vi "Window Graph.vi"(8 "error in (no error)":errorcluster, 9 "Window":dbl[unit]=10.0, 10 "Graph ref":refnum<vi>, 11 "Readable in":refnum<class "Readable.lvclass">) -> (0 "error out":errorcluster, 3 "Readable out":refnum<class "Readable.lvclass">)   [LabVIEW 2012, in "Readable.lvclass"]
uses:
  Readable.lvclass
  Readable.lvclass/Readable.ctl
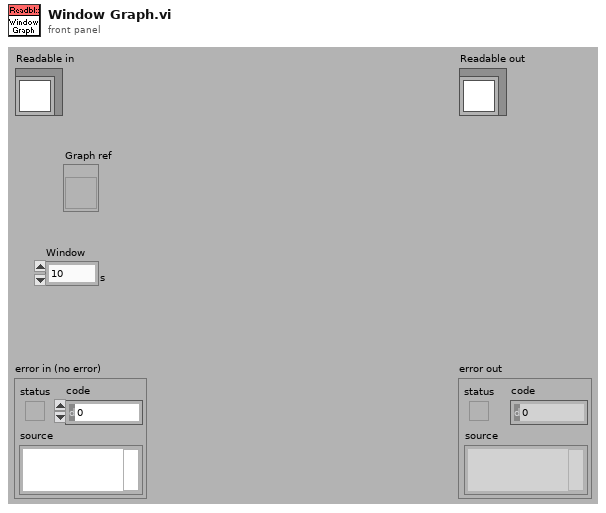
[diagram p1: front panel]
types:
  T1 = typedef "Readable.lvclass/Data Points.ctl" = T2[]
  T2 = typedef "Readable.lvclass/Data Point.ctl" = cluster{"t":T3, "x":T4}
  T3 = typedef "Readable.lvclass/Time.ctl" = timestamp
  T4 = typedef "Readable.lvclass/X.ctl" = dbl
  T5 = typedef "Readable.lvclass/Channel Units.ctl" = string[]
  T6 = typedef "Readable.lvclass/Channel Names.ctl" = string[]
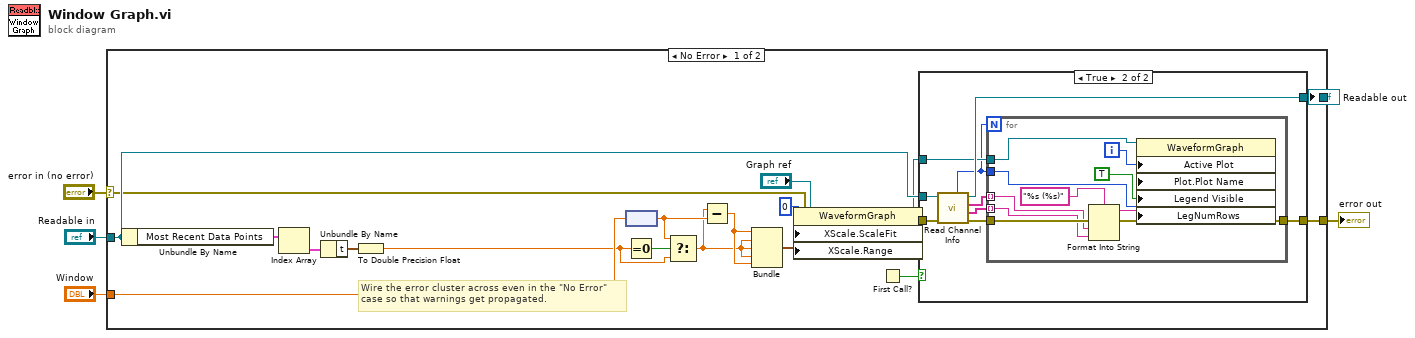
[diagram p0: block diagram]
diagram:
  n1 = case shown="No Error" "error in (no error)" {
    selector: "error in (no error)" -> [w17 w47]
    tunnel: [w8 w47] -> w4
    tunnel: [w10 w46] -> w2
    tunnel: "Readable in" -> [w24 w46]
    tunnel: "Window" -> [w18 _]
    frame No Error {
      # "Wire the error cluster across even in the \"No Error\"\ncase so that warnings get propagated."
      n2 = Unbundle By Name(w24) -> ("Most Recent Data Points"=w23:T1)
      n3 = Index Array(array=w23) -> (element=w22:T2)  [unwired: 1 in]
      n4 = Unbundle By Name(w22) -> ("t"=w21:T3)
      n5 = To Double Precision Float(number=w21) -> (double precision float=w14:dbl)
      n6 = node(w18) -> (w15:dbl)
      n7 = Equal To 0?(x=w14) -> (x = 0?=w16:bool)
      n8 = Select(t=w15, s=w16, f=w14) -> (s? t:f=w13:dbl)
      n9 = Subtract(x=w13, y=w15) -> (x-y=w20:dbl)
      n10 = Bundle(w20, w13, w13, w13, w20) -> (w12:cluster{dbl, dbl, dbl, dbl, dbl})  [unwired: 1 in]
      n11 = property on="Property Node" class="WaveformGraph"(reference="Graph ref", error in=w17, "XScale.ScaleFit"=u8 0 ("X Scale.Scale Fit"), "XScale.Range"=w12) -> (reference out=w7:refnum<vi>, error out=w9:errorcluster)
      n12 = First Call?() -> (First Call?: T/F=w6:bool)
      n13 = case shown="True" w6 {
        tunnel: w24 -> [w25 w35]
        tunnel: [w25 w34] -> w10
        tunnel: w9 -> [w26 w31]
        tunnel: [w26 w29] -> w8
        tunnel: w7 -> [_ w28]
        frame False {
        }
        frame True {
          n14 = call "Read Channel Info.vi"("error in (no error)"=w31, "Readable.lvclass in"=w35) -> ("error out"=w30:errorcluster, "Channel Units"=w32:T5, "Channel Names"=w33:T6, "Readable.lvclass out"=w34:refnum<class "Readable.lvclass">, "#Channels"=w27:i32)  [unwired: 5 in]
          n15 = for {
            N: w27 -> [_]
            tunnel: w33 -> [w42] mode=indexing
            tunnel: w30 -> [w44]
            tunnel: w32 -> [w41] mode=indexing
            tunnel: [w39] -> w29
            tunnel: w28 -> [w38]
            tunnel: w27 -> [w36]
            i -> [w45]
            n16 = Format Into String(format string="%s (%s)", error in=w44, w42, w41) -> (resulting string=w40:string, error out=w39:errorcluster)  [unwired: 1 in]
            n17 = property on="Property Node" class="WaveformGraph"(reference=w38, "Active Plot"=w45, "Plot.Plot Name"=w40, "Legend Visible"=TRUE ("Legend:Visible"), "LegNumRows"=w36) -> ()  [unwired: 1 in, 2 out]
          }
        }
      }
    }
    frame Error {
    }
  }
  "error out" <- w4
  "Readable out" <- w2
